vi "myK705.vi"(0 "run?":bool, 1 "set up\nscanner?":bool, 2 "channels":bool[](array[boolean])=[FALSE, FALSE, FALSE, FALSE, FALSE, FALSE, FALSE, FALSE, FALSE, FALSE, FALSE, FALSE, FALSE, FALSE, FALSE, FALSE, FALSE, FALSE, FALSE, FALSE], 3 "scan mode \n (step:0)":i16(slide) scale=0.0..2.0 scale format="%.2f", 4 "interval(sec)":ext=0.01 format="%.3f", 5 "last channel":ext=1.0, 6 "first channel":ext=1.0, 7 "measurement poles\n  (1-pole 20ch:0)":i16(slide) scale=0.0..2.0) -> ()   [LabVIEW 2015]
doc: "Keithley 705 Scanner\n\nUse: Allows opening a selected channel, closing the channel, scanning between a selected first and last channel, selecting scan rate and mode, and selecting 1-, 2-, or 4-pole measurement modes.\n\nDefaults: \n Measurement Poles = 1-Pole, 20 channels/card First Channel = 1\n Last channel = 1 Interval(sec) = 10mS Scan Mode = Step Channels = All channels open Trigger Mode = Internal Set Up Scanner? = No\n Run? = No\n\nAssumptions: GPIB address = 17; the bus is properly connected.\n\nCapabilities not implemented: settling time of each channel; time; date; alarm time; saving/recalling of a relay set up; SRQ.\nThese capabilities can all be implemented by adding a numeric or slide control and adding the proper command code to the command string. The codes are located on pp. 3-9 to 3-11.\n\nInteractively:\n Measurement Poles - Select a measurement-poles mode. In 2-pole operation, each channel consists of a HI and a LO line. Since there are twenty different lines on a card, 2-pole operation has a maximum of ten channels per card. In 1-pole operation, the HI and LO lines are used independently; each line is one channel. Therefore, the maximum number of channels in the 1-pole mode is twenty.\nIn 4-pole operation, each channel uses four lines, two HI and two LO lines. Thus, it requires two cards to make ten channels.\n\n Card Possible measurement-pole modes\n 7056 General Purpole Scanner 1-pole and 2-pole\n 7057 Thermocouple Scanner 2-pole\n 7058 Low Current Scanner Plug-In Card 1-pole\n\n First Channel - Select a channel from 1 to 20 to be the starting channel of a scan.\n Last Channel - Select a channel from 1 to 20 to be the ending channel in a scan. Keep in mind that the last channel can never be less than the first channel.\n Interval(sec) - Enter a time from 5mS to 999.999S. This is the time each channel is closed when using the single, continuous, or step scanning modes.\n Scan Mode - Select a scan mode.\n Channels - Select and close the desired channels.\n Trigger Mode - Select trigger mode. External trigger allows manual triggering from the front panel of the 705 via the \"START/STOP\" button or signal triggering from the rear panel via the BNC connection.\n Set Up Scanner? - Select \"Yes\" when the user wants to change the present set up parameters of the scanner. This control is implemented independently of the \"Run?\" control so that the user can use the step scan mode without resetting the scanner parameters everytime the VI is run.\n Run? - Select \"Start\" to begin a scan from the present channel when using continuous or single scan mode or to step through the next channel when using the step scan mode. Select \"Stop\" to terminate in the middle of a scan.\n\nProgrammatically: There are 8 inputs. Trigger mode is the only control that cannot be programmed. All other controls can be programmed as described below.\n\nMeasurement Poles: 0 = 1-Pole, 20 ch/card 1 = 2-Pole, 10 ch/card 2 = 4-Pole, 10 ch/card\nFirst Channel: Numeric (range 1.. 20)\nLast Channel: Numeric (range 1.. 20)\nInterval(sec): Numeric (range 5mS to 999.999S)\nScan Mode: 0 = Step Scan 1 = Single scan 2 = Cont. scan\nChannels: Bit vector (Channel 1 is at bit 1. Ignore bit 0. Keithley 705 does not have a channel 0.)\nSet up scanner?: Binary\nRun?: Binary"
panel:
  out "error out":errorcluster
  in  "error in (no error)":errorcluster
  in  "Cluster":cluster{}
  in  "trigger\nmode":bool
  # "KEITHLEY 705 SCANNER"
  # "yes\n\nno"
  # "close\nopen"
  # "start\n\nstop"
  # "ext\nint"
  # "© Copyright 1993 National Instruments Corporation.  All Rights Reserved."
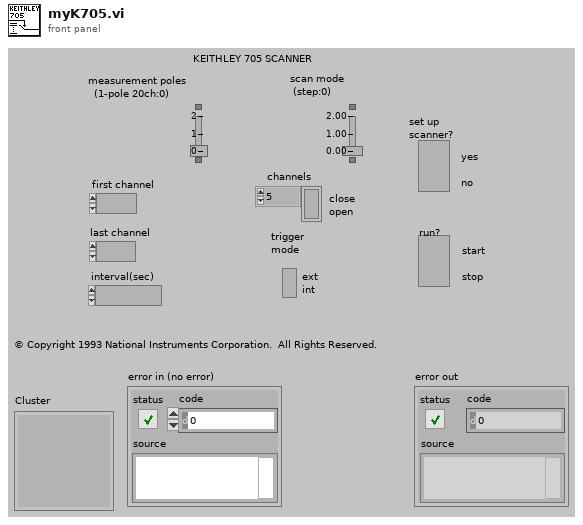
[diagram p1: front panel]
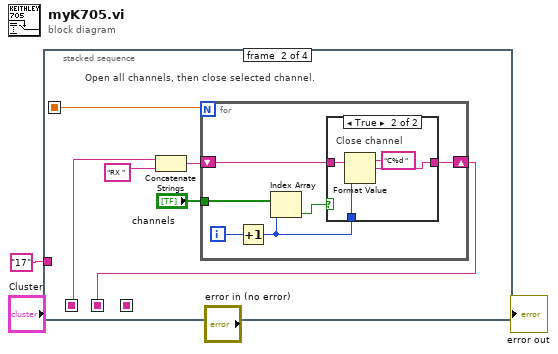
[diagram p0: block diagram]
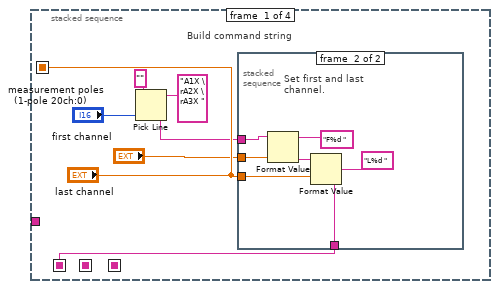
[diagram p2: hidden frame]
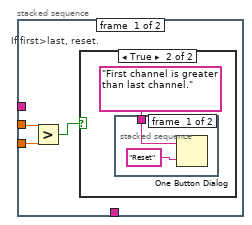
[diagram p3: hidden frame]
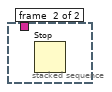
[diagram p5: hidden frame]
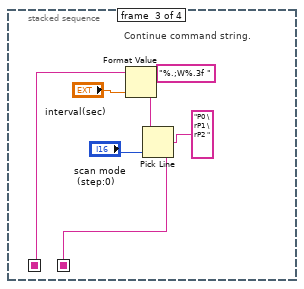
[diagram p7: hidden frame]
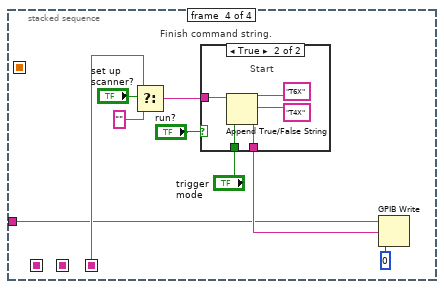
[diagram p8: hidden frame]
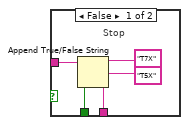
[diagram p9: hidden frame]
diagram:
  n1 = stacked-sequence {
    seq-local: [w5 _ _ _] -> [_ w24 _ _]
    seq-local: [_ w27 _ _] -> [_ _ w44 _]
    seq-local: [_ _ w45 _] -> [_ _ _ w48]
    seq-local: ["last channel" _ _ _] -> [_ w22 _ _]
    tunnel: "17" -> [_ _ _ w46]
    frame #0 {
      # "Build command string"
      n2 = Pick Line(string ("")="", multi-line string="A1X \rA2X \rA3X ", line index="measurement poles\n  (1-pole 20ch:0)") -> (output string=w4:string)
      n3 = stacked-sequence {
        tunnel: w4 -> [_ w15]
        tunnel: "first channel" -> [w9 w17]
        tunnel: "last channel" -> [w10 w18]
        tunnel: [_ w21] -> w5
        frame #0 {
          # "If first>last, reset."
          n4 = Greater?(x=w9, y=w10) -> (0:w11:bool)
          n5 = case shown="True" w11 {
            frame False {
            }
            frame True {
              n6 = stacked-sequence {
                tunnel: "First channel is greater than last channel." -> [w13 _]
                frame #0 {
                  n7 = One Button Dialog(message=w13, button name ("OK")="Reset") -> ()  [unwired: 1 out]
                }
                frame #1 {
                  n8 = Stop() -> ()  [unwired: 1 in]
                }
              }
            }
          }
        }
        frame #1 {
          # "Set first and last\nchannel."
          n9 = Format Value(string ("")=w15, format string="F%d ", value (0)=w17) -> (output string=w19:string)
          n10 = Format Value(string ("")=w19, format string="L%d ", value (0)=w18) -> (output string=w21:string)
        }
      }
    }
    frame #1 {
      # "Open all channels, then close selected channel."
      n11 = Concatenate Strings(w24, "RX ") -> (w26:string)
      n12 = for {
        N: w22 -> [_]
        shift-right: [w33] -> w27
        shift-left: w26 -> [w32]
        tunnel: "channels" -> [w29]
        i -> [w28]
        n13 = Increment(x=w28) -> (x+1=w31:i32)
        n14 = Index Array(array=w29, index=w31) -> (element=w30:bool)
        n15 = case shown="True" w30 {
          tunnel: w32 -> [w34 w35]
          tunnel: w31 -> [_ w36]
          tunnel: [w34 w38] -> w33
          frame False {
            # "Leave channel\n    open"
          }
          frame True {
            # "Close channel"
            n16 = Format Value(string ("")=w35, format string="C%d ", value (0)=w36) -> (output string=w38:string)
          }
        }
      }
    }
    frame #2 {
      # "Continue command string."
      n17 = Format Value(string ("")=w44, format string="%.;W%.3f ", value (0)="interval(sec)") -> (output string=w41:string)
      n18 = Pick Line(string ("")=w41, multi-line string="P0 \rP1 \rP2 ", line index="scan mode \n (step:0)") -> (output string=w45:string)
    }
    frame #3 {
      # "Finish command string."
      n19 = Select(t=w48, s="set up\nscanner?", f="") -> (s? t:f=w52:string)
      n20 = case shown="True" "run?" {
        tunnel: w52 -> [w55 w60]
        tunnel: "trigger\nmode" -> [w56 w64]
        tunnel: [w59 w63] -> w54
        frame False {
          # "Stop"
          n21 = Append True/False String(1:w56, 2:"T5X", 3:"T7X", 4:w55) -> (0:w59:string)
        }
        frame True {
          # "Start"
          n22 = Append True/False String(1:w64, 2:"T4X", 3:"T6X", 4:w60) -> (0:w63:string)
        }
      }
      n23 = GPIB Write(0:w46, 1:w54, 2:0) -> ()  [unwired: 2 in, 2 out]
    }
  }
